vi "Init.vi"(8 "error in (no error)":errorcluster, 10 "Address":string, 11 "ArduinoTranslationStage in":refnum<class "ArduinoTranslationStage.lvclass">) -> (0 "error out":errorcluster, 3 "ArduinoTranslationStage out":refnum<class "ArduinoTranslationStage.lvclass">)   [LabVIEW 2023, in "ArduinoTranslationStage.lvlib" / "ArduinoTranslationStage.lvclass"]
uses:
  ArduinoTranslationStage.lvclass
  typedefs/instrumentType.ctl
  <vilib>/Instr/_visa.llb/Select Event Type.ctl
  ArduinoTranslationStage.lvclass/ArduinoTranslationStage.ctl
  <vilib>/ActorFramework/Actor/Actor.lvclass/Actor.ctl
  Interfaces/InitDeinitInterface/InitDeinitComm Messages/InitDone Msg/InitDone Msg.lvclass/InitDone Msg.ctl
  <vilib>/ActorFramework/Message Enqueuer/Message Enqueuer.lvclass/Message Enqueuer.ctl
  <vilib>/ActorFramework/Message Enqueuer/Enqueue.vi
  Interfaces/InitDeinitInterface/InitDeinitComm Messages/InitDone Msg/InitDone Msg.lvclass
  <vilib>/ActorFramework/Message Priority Queue/Priority Enqueue.vi
  <vilib>/ActorFramework/Actor/Actor.lvclass
  typedefs/typedefs.lvlib
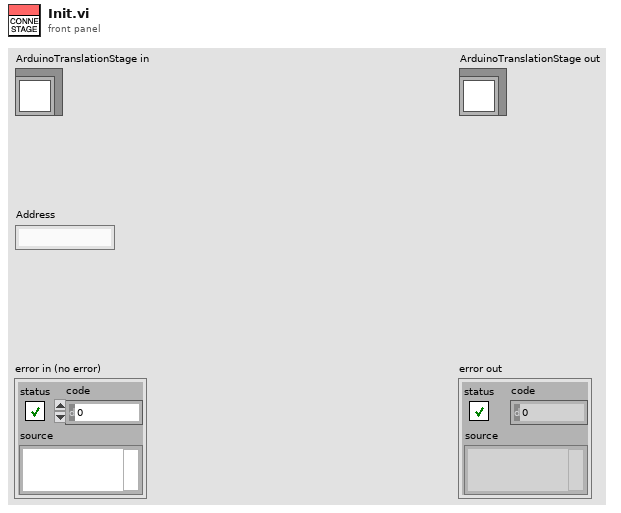
[diagram p1: front panel]
types:
  T1 = typedef "typedefs.lvlib/instrumentType.ctl" = enum16{"Spectrometer", "Camera", "Stepper", "Piezo", "SLM"}
  T2 = typedef "Select Event Type.ctl" = u32
  T3 = cluster{"address type":enum16{"VISA", "Index"}, "Address":string, "instrument type":T1}
  T4 = cluster{"Instr Error":errorcluster, "Stepper Data":cluster{"Channel Count":i32}, "Address":cluster{"address type":enum16{"VISA", "Index"}, "Address":string, "instrument type":T1}}
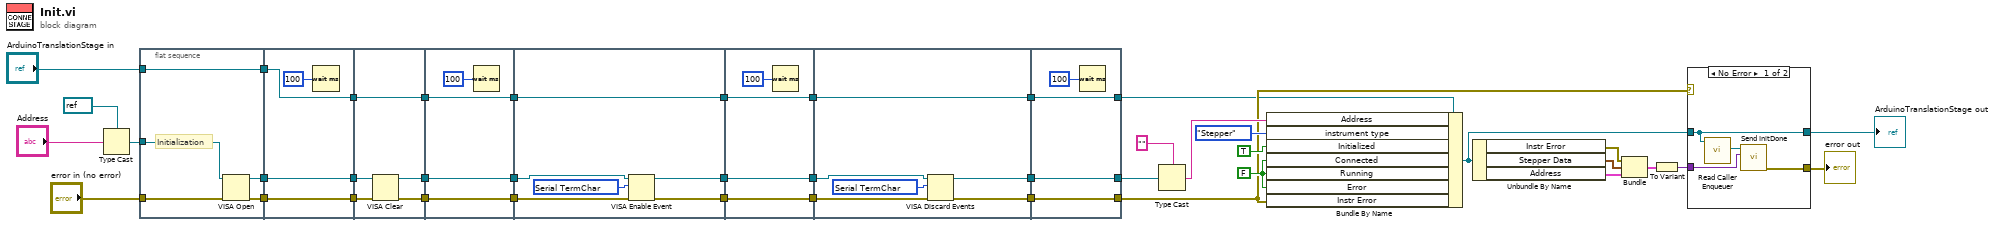
[diagram p0: block diagram]
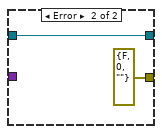
[diagram p2: hidden frame]
diagram:
  w28 = FALSE ("InstrumentData.CurrentState.Connected")
  n1 = Type Cast(type=refnum<visa-resource-name> refnum ("VISA resource name"), x="Address") -> (*(type *) &x=w34:refnum<visa-resource-name>)
  n2 = flat-sequence {
    tunnel: [w47] -> w42
    tunnel: [w46] -> w41
    tunnel: w34 -> [w45]
    tunnel: "error in (no error)" -> [w44]
    tunnel: [w43] -> w9
    tunnel: "ArduinoTranslationStage in" -> [w43]
    tunnel: [w50] -> w40
    tunnel: w42 -> [w50]
    tunnel: [w49] -> w39
    tunnel: w41 -> [w49]
    tunnel: [w48] -> w10
    tunnel: w9 -> [w48]
    tunnel: [w54] -> w38
    tunnel: [w53] -> w37
    tunnel: w40 -> [w56]
    tunnel: w39 -> [w55]
    tunnel: [w52] -> w11
    tunnel: w10 -> [w52]
    tunnel: w38 -> [w60]
    tunnel: w37 -> [w59]
    tunnel: [w60] -> w27
    tunnel: [w59] -> w26
    tunnel: [w57] -> w12
    tunnel: w11 -> [w57]
    tunnel: w27 -> [w65]
    tunnel: w26 -> [w66]
    tunnel: [w63] -> w24
    tunnel: [w62] -> w21
    tunnel: [w61] -> w13
    tunnel: w12 -> [w61]
    tunnel: [w69] -> w25
    tunnel: w24 -> [w69]
    tunnel: w21 -> [w68]
    tunnel: [w68] -> w20
    tunnel: [w67] -> w14
    tunnel: w13 -> [w67]
    tunnel: w25 -> [w76]
    tunnel: [w75] -> w22
    tunnel: w20 -> [w74]
    tunnel: [w73] -> w19
    tunnel: [w72] -> w15
    tunnel: w14 -> [w72]
    tunnel: [w79] -> w23
    tunnel: w22 -> [w79]
    tunnel: w19 -> [w78]
    tunnel: [w78] -> w18
    tunnel: [w77] -> w16
    tunnel: w15 -> [w77]
    frame #0 {
      # "Initialization"
      n3 = VISA Open(error in (no error)=w44, VISA resource name=w45) -> (VISA resource name=w46:refnum<visa-resource-name>, error out=w47:errorcluster)  [unwired: 3 in]
    }
    frame #1 {
      n4 = Wait (ms)(milliseconds to wait=u32 100) -> ()  [unwired: 1 out]
    }
    frame #2 {
      n5 = VISA Clear(VISA resource name=w55, error in (no error)=w56) -> (VISA resource name out=w53:refnum<visa-resource-name>, error out=w54:errorcluster)
    }
    frame #3 {
      n6 = Wait (ms)(milliseconds to wait=u32 100) -> ()  [unwired: 1 out]
    }
    frame #4 {
      w64 = T2 1073684516 items=["Service Request"=1073684491, "Trigger"=3221168138, "Clear"=1073684493, "VXI Signal"=1073684512, "VXI/VME Interrupt"=3221168161, "VXI/VME Sysfail"=1073684509, "VXI/VME Sysreset"=1073684510, "GPIB CIC"=1073684498, "GPIB Talk"=1073684499, "GPIB Listen"=1073684500, "PXI Interrupt"=1073684514, "Serial Break"=1073684515, "Serial TermChar"=1073684516, "Serial CTS"=1073684521, "Serial DSR"=1073684522, "Serial DCD"=1073684524, "Serial RI"=1073684526, "Serial Character"=1073684533, "USB Interrupt"=1073684535, "All Enabled"=1073709055] ("Event Type")
      n7 = VISA Enable Event(8:w65, 10:w64, 11:w66) -> (0:w62:errorcluster, 3:w63:refnum<visa-resource-name>)  [unwired: 1 in]
    }
    frame #5 {
      n8 = Wait (ms)(milliseconds to wait=u32 100) -> ()  [unwired: 1 out]
    }
    frame #6 {
      w71 = T2 1073684516 items=["Service Request"=1073684491, "Trigger"=3221168138, "Clear"=1073684493, "VXI Signal"=1073684512, "VXI/VME Interrupt"=3221168161, "VXI/VME Sysfail"=1073684509, "VXI/VME Sysreset"=1073684510, "GPIB CIC"=1073684498, "GPIB Talk"=1073684499, "GPIB Listen"=1073684500, "PXI Interrupt"=1073684514, "Serial Break"=1073684515, "Serial TermChar"=1073684516, "Serial CTS"=1073684521, "Serial DSR"=1073684522, "Serial DCD"=1073684524, "Serial RI"=1073684526, "Serial Character"=1073684533, "USB Interrupt"=1073684535, "All Enabled"=1073709055] ("Event Type")
      n9 = VISA Discard Events(8:w74, 10:w71, 11:w76) -> (0:w73:errorcluster, 3:w75:refnum<visa-resource-name>)  [unwired: 1 in]
    }
    frame #7 {
      n10 = Wait (ms)(milliseconds to wait=u32 100) -> ()  [unwired: 1 out]
    }
  }
  n11 = Type Cast(type="", x=w23) -> (*(type *) &x=w31:string)
  n12 = Bundle By Name(cluster=w16, "Address"=w31, "instrument type"=instrumentType."Stepper" ("InstrumentData.Address.instrument type"), "Initialized"=TRUE ("InstrumentData.CurrentState.Initialized"), "Connected"=w28, "Running"=w28, "Error"=w28, "Instr Error"=w18) -> (w3:refnum<class "ArduinoTranslationStage.lvclass">)
  n13 = Unbundle By Name(w3) -> ("Instr Error"=w4:errorcluster, "Stepper Data"=w5:cluster{"Channel Count":i32}, "Address"=w6:T3)
  n14 = Bundle("Instr Error"=w4, "Stepper Data"=w5, "Address"=w6) -> (w1:T4)  [unwired: 1 in]
  n15 = To Variant(anything=w1) -> (Variant=w2:variant)
  n16 = case shown="No Error" w18 {
    tunnel: w3 -> [w83 w86]
    tunnel: [w83 w86] -> w17
    tunnel: [w82 errorcluster {"status"=FALSE, "code"=0, "source"=""} ("error out")] -> w7
    tunnel: w2 -> [w81 _]
    frame No Error {
      n17 = call <vilib>:"Read Caller Enqueuer.vi"("Actor"=w83) -> ("Caller Enqueuer"=w84:refnum<class "Message Enqueuer.lvclass">)  [unwired: 10 in]
      n18 = call "Send InitDone.vi"("Variant"=w81, "Message Enqueuer"=w84) -> ("error out"=w82:errorcluster)  [unwired: 8 in, 1 out]
    }
    frame Error {
    }
  }
  "error out" <- w7
  "ArduinoTranslationStage out" <- w17
